vi "Destroy Stream Endpoint.vi"(8 "error in (no error)":errorcluster, 11 "Refnum in":refnum<k21>) -> (0 "error out":errorcluster)   [LabVIEW 2011]
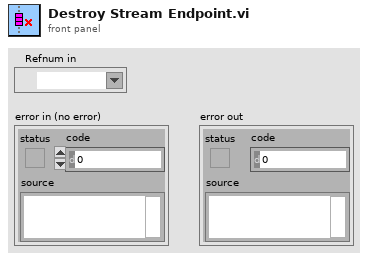
[diagram p1: front panel]
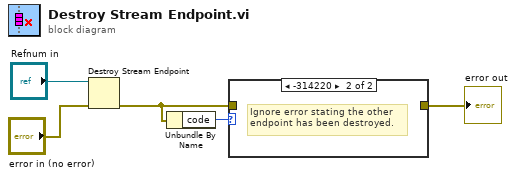
[diagram p0: block diagram]
diagram:
  n1 = Destroy Stream Endpoint(8:"error in (no error)", 11:"Refnum in") -> (0:w4:errorcluster)
  n2 = Unbundle By Name(w4) -> ("code"=w3:i32)
  n3 = case shown="-314220" w3 {
    tunnel: w4 -> [w6 _]
    tunnel: [w6 _] -> w5
    frame 0, Default {
    }
    frame -314220 {
      # "Ignore error stating the other\nendpoint has been destroyed."
    }
  }
  "error out" <- w5
